vi "RT Driver VI.vi"(6 "Device Clock":string, 9 "Device Inputs FIFO":refnum<k33>, 10 "Device Outputs FIFO":refnum<k33>, 11 "Device Reference":T1 format="%.0x") -> ()   [LabVIEW 2019, in "Displacement Measurement CD Engine.lvlib"]
uses:
  Displacement Measurement CD Engine.lvlib
  <vilib>/NI VeriStand/Custom Device API/Custom Device Item Ref.ctl
  <vilib>/NI VeriStand/Custom Device API/Custom Device Channel Type.ctl
  <vilib>/NI VeriStand/Custom Device API/Message Response (String).ctl
  <vilib>/NI VeriStand/Custom Device API/Message Response (Byte Array).ctl
  <vilib>/DAQmx/read.llb/DAQmx Read (Analog 2D DBL NChan NSamp).vi
  <vilib>/NI VeriStand/Custom Device API/Get Item Property (Double).vi
  <vilib>/NI VeriStand/Custom Device API/Get Item Property (String).vi
  <vilib>/DAQmx/create/channels.llb/DAQmx Create Channel (AI-Voltage-Basic).vi
  <vilib>/DAQmx/configure/timing.llb/DAQmx Timing (Sample Clock).vi
  <vilib>/DAQmx/miscellaneous.llb/DAQmx Fill In Error Info.vi
  <vilib>/NI VeriStand/Custom Device API/Custom Device API.lvlib
  <vilib>/NI VeriStand/Custom Device Tools/Custom Device Utility Library/Custom Device Utility Library.lvlib
  <resource>/objmgr/daqmx.rc
panel:
  in  "Initialization Status Notifier":refnum<notifier>
  in  "Status Notifier":refnum<notifier>
  # "Custom Device Template\nv1.0"
  # "Use this template as a starting point for creating a custom device code module. The input controls shown here are specially named controls that the system will use to provide the device loop with data. The controls are not required for the device loop to run. For instance, if the device doesn't produce any output data, then you don't need the Device Outputs FIFO control. If you do use these controls, however, they need to have these exact names to be functional."
  # "The optional status notifier element is used to notify the RT engine of the last state of the custom device, and to indicate the device has completed execution. If this control is not used, a default No Error value is returned to the system when the device finishes execution.\n\nNote: This error state is not checked until the system shuts down. Use an output status channel to send more immediate status values to the system."
  # "This optional input can be used to send the VeriStand Engine the final status of the custom device initalization process. If this control exists on the custom device front panel, the VeriStand Engine will wait for a status update before starting up. If the custom device reports an error, that will abort the execution of the current configuration in the VeriStand Engine.\n\nThis control can be deleted if the custom device does not need to send the initialization status update."
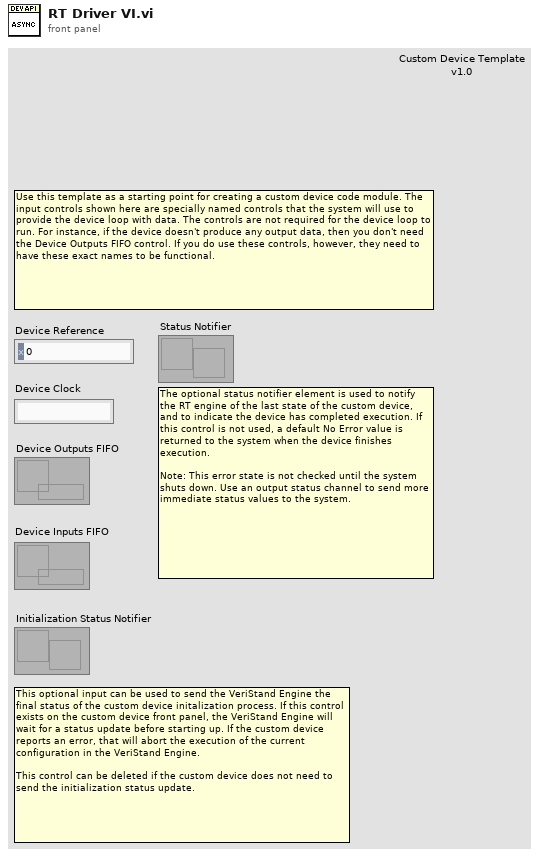
[diagram p1: front panel]
types:
  T1 = typedef "Custom Device API.lvlib/Custom Device Item Ref.ctl" = u64
  T2 = typedef "Custom Device API.lvlib/Custom Device Channel Type.ctl" = enum16{"Input", "Output"}
  T3 = typedef "Custom Device API.lvlib/Custom Device Engine Event Ref.ctl" = refnum<event-registration>
  T4 = typedef "Custom Device API.lvlib/Message Response (String).ctl" = cluster{"Response":string, "Error":errorcluster}
  T5 = typedef "Custom Device API.lvlib/Message Response (Byte Array).ctl" = cluster{"Response":u8[], "Error":errorcluster}
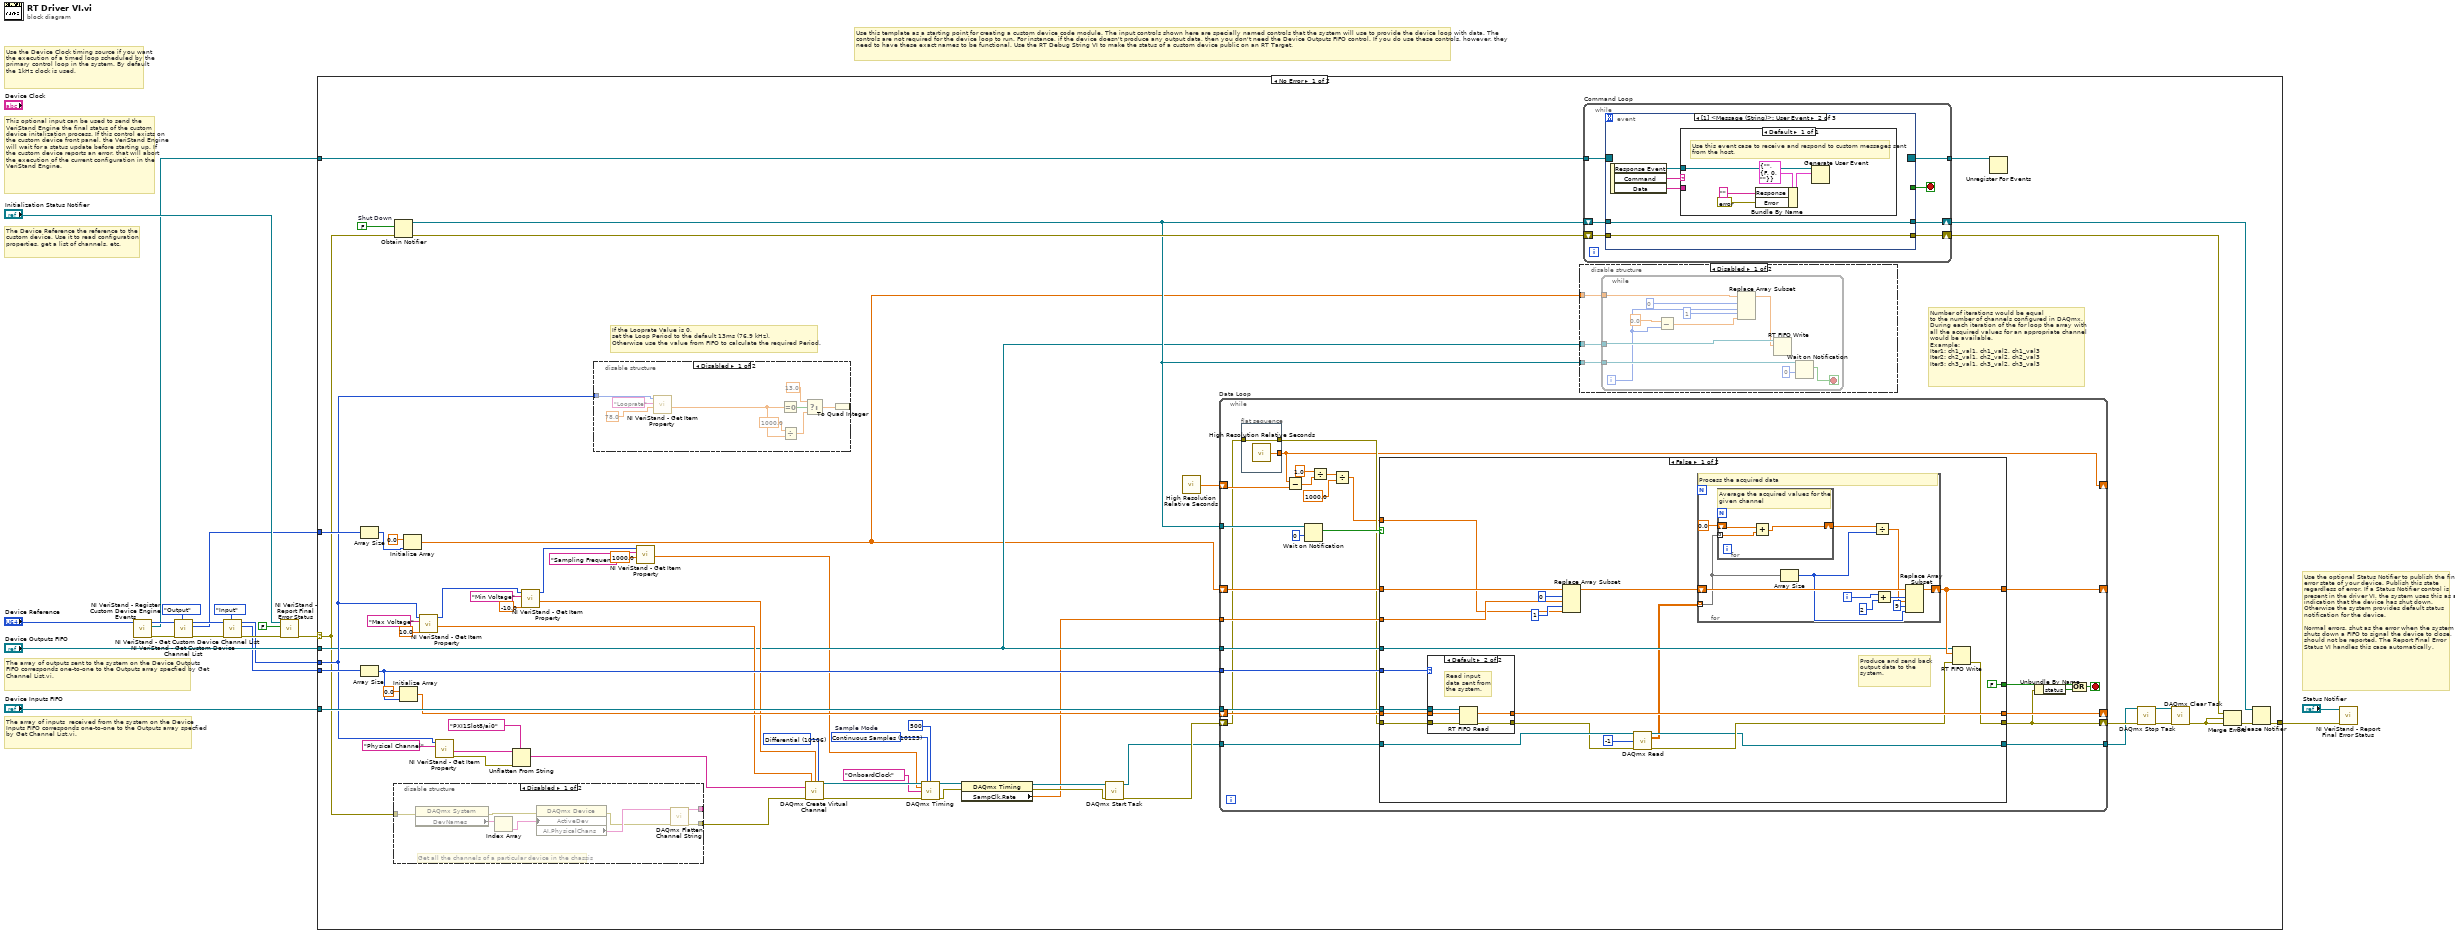
[diagram p0: block diagram]
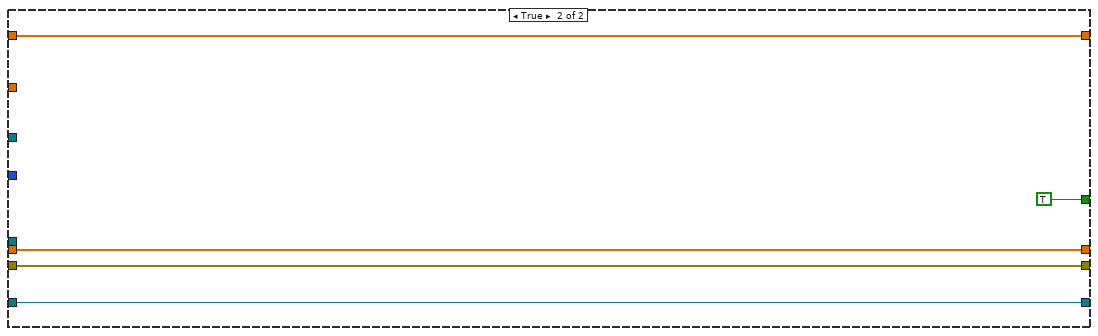
[diagram p4: hidden frame]
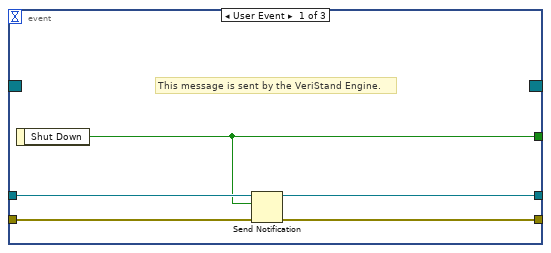
[diagram p7: hidden frame]
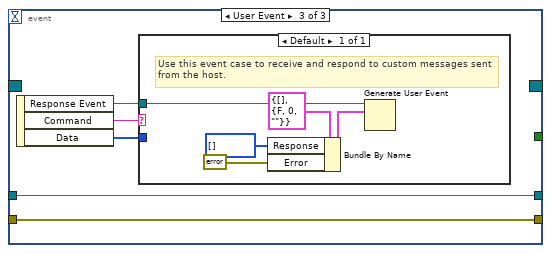
[diagram p8: hidden frame]
diagram:
  # "This optional input can be used to send the VeriStand Engine the final status of the custom device initalization process. If this control exists on the custom device front panel, the VeriStand Engine will wait for a status update before starting up. If the custom device reports an error, that will abort the execution of the current configuration in the VeriStand Engine."
  # "The array of inputs  received from the system on the Device Inputs FIFO corresponds one-to-one to the Outputs array specfied by Get Channel List.vi."
  # "Use the optional Status Notifier to publish the final error state of your device. Publish this state regardless of error. If a Status Notifier control is present in the driver VI, the system uses this as an indication that the device has shut down. Otherwise the system provides default status notification for the device.\n\nNormal errors, shut as the error when the system shuts down a FIFO to signal the device to close, should not be reported. The Report Final Error Status VI handles this case automatically."
  # "The array of outputs sent to the system on the Device Outputs FIFO corresponds one-to-one to the Outputs array specfied by Get Channel List.vi."
  # "The Device Reference the reference to the custom device. Use it to read configuration properties, get a list of channels, etc."
  # "Use the Device Clock timing source if you want the execution of a timed loop scheduled by the primary control loop in the system. By default the 1kHz clock is used."
  # "Use this template as a starting point for creating a custom device code module. The input controls shown here are specially named controls that the system will use to provide the device loop with data. The controls are not required for the device loop to run. For instance, if the device doesn't produce any output data, then you don't need the Device Outputs FIFO control. If you do use these controls, however, they need to have these exact names to be functional. Use the RT Debug String VI to make the status of a custom device public on an RT Target."
  n1 = call <vilib>:"NI VeriStand - Register Custom Device Engine Events.vi"("Device Ref in"="Device Reference") -> ("error out"=w19:errorcluster, "Custom Device Engine Event Ref"=w4:T3, "Device Ref out"=w10:T1)  [unwired: 8 in]
  n2 = call <vilib>:"NI VeriStand - Get Custom Device Channel List.vi"("Channel Type"=Custom_Device_Channel_Type."Output", "error in (no error)"=w19, "Device Ref in"=w10) -> ("error out"=w14:errorcluster, "Specified Channel Ref List"=w3:T1[], "Device Ref out"=w15:T1)  [unwired: 6 out]
  n3 = call <vilib>:"NI VeriStand - Get Custom Device Channel List.vi"("Channel Type"=Custom_Device_Channel_Type."Input", "error in (no error)"=w14, "Device Ref in"=w15) -> ("error out"=w18:errorcluster, "Specified Channel Ref List"=w6:T1[], "Device Ref out"=w2:T1)  [unwired: 6 out]
  n4 = call <vilib>:"NI VeriStand - Report Final Error Status.vi"("error in (no error)"=w18, "Filter FIFO & Shutdown Errors (T)"=FALSE ("Filter FIFO Errors (T)"), "Status Notifier"="Initialization Status Notifier") -> ("error out"=w1:errorcluster)  [unwired: 8 out]
  n5 = case shown="No Error" w1 {
    selector: w1 -> [w28 w215]
    tunnel: "Device Outputs FIFO" -> [w34 _]
    tunnel: "Device Inputs FIFO" -> [w75 _]
    tunnel: w6 -> [w71 _]
    tunnel: w3 -> [w70 _]
    tunnel: w4 -> [w68 _]
    tunnel: [w66 w215] -> w5
    tunnel: w2 -> [w43 _]
    frame No Error {
      w49 = 10106 items=["default"=-1, "RSE"=10083, "NRSE"=10078, "Differential"=10106, "Pseudodifferential"=12529] ("Terminal Configuration")
      w51 = 10123 items=["Finite Samples"=10178, "Continuous Samples"=10123, "Hardware Timed Single Point"=12522]  # Sample Mode
      w67 = FALSE  # Shut Down
      # "Number of iterations would be equal\nto the number of channels configured in DAQmx.\nDuring each iteration of the for loop the array with\nall the acquired values for an appropriate channel\nwould be available.\nExample:\nIter1: ch1_val1, ch1_val2, ch1_val3\nIter2: ch2_val1, ch2_val2, ch2_val3\nIter3: ch3_val1, ch3_val2, ch3_val3"
      # "If the Looprate Value is 0,\nset the Loop Period to the default 13ms (76.9 kHz).\nOtherwise use the value from FIFO to calculate the required Period."
      n6 = Array Size(array=w71) -> (size(s)=w69:i32)
      n7 = Array Size(array=w70) -> (size(s)=w72:i32)
      n8 = disable-structure shown="Disabled" {
        disable-tunnel: [w166 _] -> _
        disable-tunnel: w28 -> [w164 _]
        disable-tunnel: [w161 _] -> w27
        frame Disabled {
          # "Get all the channels of a particular device in the chassis"
          n9 = property class="DAQmx System"(error in=w164) -> (error out=w163:errorcluster, "DevNames"=w168:tag[])  [unwired: 1 in, 1 out]
          n10 = Index Array(array=w168) -> (element=w167:tag)  [unwired: 1 in]
          n11 = property class="DAQmx Device"(error in=w163, "ActiveDev"=w167) -> (error out=w162:errorcluster, "AI.PhysicalChans"=w165:tag[])  [unwired: 1 in, 1 out]
          n12 = call <vilib>:"DAQmx Flatten Channel String.vi"("names in"=w165, "error in"=w162) -> ("names out"=w166:string, "error out"=w161:errorcluster)  [unwired: 12 in]
        }
        frame Enabled {
        }
      }
      n13 = Obtain Notifier(notification data type=w67, error in (no error)=w28) -> (notifier out=w35:refnum<notifier>, error out=w76:errorcluster)  [unwired: 2 in, 1 out]
      n14 = Initialize Array(0.0 ("element"), w69) -> (w62:dbl[])
      n15 = Initialize Array(0.0 ("element"), w72) -> (w33:dbl[])
      n16 = call-poly <vilib>:"NI VeriStand - Get Item Property.vi"("Default Value"=10.0, "Property Name"="Max Voltage", "Item Ref in"=w43) -> ("Value"=w41:dbl, "Item Ref out"=w42:T1)  [unwired: 5 in, 2 out]
      n17 = call-poly <vilib>:"NI VeriStand - Get Item Property.vi"("Property Name"="Physical Channel", "Item Ref in"=w43) -> ("error out"=w45:errorcluster, "Value"=w29:string)  [unwired: 6 in, 2 out]
      n18 = Unflatten From String(type=tag "PXI1Slot8/ai0" ("Physical Channel"), binary string=w29, error in (no error)=w45) -> (value=w24:tag)  [unwired: 2 in, 2 out]
      n19 = call-poly <vilib>:"NI VeriStand - Get Item Property.vi"("Default Value"=-10.0, "Property Name"="Min Voltage", "Item Ref in"=w42) -> ("Value"=w40:dbl, "Item Ref out"=w44:T1)  [unwired: 5 in, 2 out]
      n20 = disable-structure shown="Disabled" {
        disable-tunnel: w43 -> [w79 _]
        frame Disabled {
          n21 = call-poly <vilib>:"NI VeriStand - Get Item Property.vi"("Default Value"=78.0, "Property Name"="Looprate", "Item Ref in"=w79) -> ("Value"=w77:dbl)  [unwired: 5 in, 3 out]
          n22 = Equal To 0?(x=w77) -> (x = 0?=w84:bool)
          n23 = Divide(x=1000.0, y=w77) -> (x/y=w82:dbl)
          n24 = Select(t=13.0, s=w84, f=w82) -> (s? t:f=w81:dbl)
          n25 = To Quad Integer(1:w81) -> ()  [unwired: 1 out]
        }
        frame Enabled {
        }
      }
      n26 = call-poly <vilib>:"NI VeriStand - Get Item Property.vi"("Default Value"=1000.0, "Property Name"="Sampling Frequency", "Item Ref in"=w44) -> ("Value"=w23:dbl)  [unwired: 5 in, 3 out]
      n27 = call-poly <vilib>:"DAQmx Create Virtual Channel.vi"("maximum value"=w41, "minimum value"=w40, "input terminal configuration"=w49, "physical channels"=w24, "error in"=w27) -> ("task out"=w50:refnum<k21>, "error out"=w30:errorcluster)  [unwired: 9 in]
      n28 = call-poly <vilib>:"DAQmx Timing.vi"("task/channels in"=w50, "sample mode"=w51, "samples per channel"=500, "rate"=w23, "source"=tag "OnboardClock" ("Sample Clock Source"), "error in"=w30) -> ("task out"=w53:refnum<k21>, "error out"=w52:errorcluster)  [unwired: 8 in]
      n29 = property class="DAQmx Timing"(reference=w53, error in=w52) -> (reference out=w47:refnum<k21>, error out=w46:errorcluster, "SampClk.Rate"=w22:dbl)
      n30 = call <vilib>:"DAQmx Start Task.vi"("task/channels in"=w47, "error in"=w46) -> ("task out"=w25:refnum<k21>, "error out"=w26:errorcluster)  [unwired: 12 in]
      n31 = call <vilib>:"High Resolution Relative Seconds.vi"() -> ("relative seconds"=w21:dbl)
      n32 = while "Data Loop" {
        shift-right: [w110] -> _
        shift-left: w62 -> [w111]
        shift-right: [w105] -> w59
        shift-left: w26 -> [w93]
        shift-right: [w109] -> _
        shift-left: w33 -> [w97]
        tunnel: w34 -> [w96]
        tunnel: w75 -> [w108]
        tunnel: w69 -> [w107]
        tunnel: w35 -> [w104]
        tunnel: w25 -> [w99]
        tunnel: [w98] -> w58
        tunnel: w22 -> [w95]
        shift-right: [w91] -> _
        shift-left: w21 -> [w94]
        stop <- w100 stop-if-true
        n33 = flat-sequence {
          tunnel: w93 -> [w113]
          tunnel: [w113] -> w92
          tunnel: [w112] -> w91
          frame #0 {
            n34 = call <vilib>:"High Resolution Relative Seconds.vi"() -> ("relative seconds"=w112:dbl)
          }
        }
        n35 = Subtract(x=w91, y=w94) -> (x-y=w89:dbl)
        n36 = Wait on Notification(notifier=w104, timeout in ms (-1)=0) -> (notification=w103:bool)  [unwired: 2 in, 3 out]
        n37 = Divide(x=1.0, y=w89) -> (x/y=w88:dbl)
        n38 = Divide(x=w88, y=1000.0) -> (x/y=w86:dbl)
        n39 = case shown="False" w103 {
          tunnel: w92 -> [w134 w159]
          tunnel: w111 -> [w133 w160]
          tunnel: [w132 w160] -> w110
          tunnel: w97 -> [w122 w158]
          tunnel: [w119 w158] -> w109
          tunnel: w96 -> [w118 _]
          tunnel: w108 -> [w131 _]
          tunnel: w107 -> [w130 _]
          tunnel: [w129 w159] -> w105
          tunnel: [FALSE TRUE] -> w101
          tunnel: w99 -> [w128 w156]
          tunnel: [w125 w156] -> w98
          tunnel: w95 -> [w117 _]
          tunnel: w86 -> [w115 _]
          frame False {
            # "Produce and send back output data to the system."
            n40 = case shown="Default" w130 {
              tunnel: w131 -> [_ w155]
              tunnel: w133 -> [w150 w154]
              tunnel: [w150 w153] -> w132
              tunnel: [w149 w152] -> w127
              tunnel: w134 -> [w149 w151]
              frame 0 {
                # "No inputs to read\nfrom system. Inputs FIFO not created in this case, so don't write to it."
              }
              frame Default {
                # "Read input data sent from the system."
                n41 = RT FIFO Read(0:w155, 1:w154, 3:w151) -> (9:w153:dbl[], 11:w152:errorcluster)  [unwired: 4 out]
              }
            }
            n42 = Replace Array Subset(array=w122, new element #1=w117, index #1=0 ("index"), new element #2=w115, index #2=1 ("index")) -> (w120:dbl[])
            n43 = call-poly <vilib>:"DAQmx Read.vi"("task/channels in"=w128, "number of samples per channel"=-1, "error in"=w127) -> ("task out"=w125:refnum<k21>, "data"=w114:dbl[][], "error out"=w126:errorcluster)  [unwired: 10 in]
            n44 = for {
              shift-right: [w144] -> w119
              shift-left: w120 -> [w145]
              tunnel: w114 -> [w137] mode=indexing
              i -> [w143]
              # "Process the acquired data"
              n45 = for {
                tunnel: w137 -> [w147] mode=indexing
                shift-right: [w146] -> w139
                shift-left: 0.0 -> [w148]
                # "Average the acquired values for the given channel"
                n46 = Add(x=w148, y=w147) -> (x+y=w146:dbl)
              }
              n47 = Array Size(array=w137) -> (size(s)=w135:i32)
              n48 = Divide(x=w139, y=w135) -> (x/y=w138:dbl)
              n49 = Add(x=w143, y=2) -> (x+y=w141:i32)
              n50 = Replace Array Subset(array=w145, new element #1=w138, index #1=w141, new element #2=w135, index #2=9 ("index")) -> (w144:dbl[])
            }
            n51 = RT FIFO Write(0:w118, 1:w119, 3:w126) -> (11:w129:errorcluster)  [unwired: 1 in, 4 out]
          }
          frame True {
          }
        }
        n52 = Unbundle By Name(w105) -> ("status"=w102:bool)
        n53 = Compound Arithmetic op=OR(w101, w102) -> (w100:bool)
      }
      n54 = disable-structure shown="Disabled" {
        disable-tunnel: w35 -> [w171 _]
        disable-tunnel: w34 -> [w170 _]
        disable-tunnel: w33 -> [w169 _]
        frame Disabled {
          n55 = while {
            tunnel: w171 -> [w180]
            tunnel: w170 -> [w179]
            tunnel: w169 -> [w177]
            i -> [w174]
            stop <- w181 stop-if-true
            n56 = Subtract(x=0.0, y=w174) -> (x-y=w173:dbl)
            n57 = Replace Array Subset(array=w177, new element #1=w174, index #1=0 ("index"), new element #2=w173, index #2=1 ("index")) -> (w176:dbl[])
            n58 = RT FIFO Write(0:w179, 1:w176) -> ()  [unwired: 2 in, 5 out]
            n59 = Wait on Notification(notifier=w180, timeout in ms (-1)=0) -> (notification=w181:bool)  [unwired: 2 in, 3 out]
          }
        }
        frame Enabled {
        }
      }
      n60 = while "Command Loop" {
        tunnel: w68 -> [w189]
        tunnel: [w188] -> w65
        shift-right: [w185] -> w64
        shift-left: w35 -> [w186]
        shift-right: [w183] -> w39
        shift-left: w76 -> [w184]
        stop <- w187 stop-if-true
        n61 = event shown="[1] <Message (String)>: User Event" {
          selector: w189 -> [_ _ _]
          dyn-events: [_ _ _] -> w188
          timeout: _ -> [_ _ _]
          tunnel: [w192 _ _] -> w187
          tunnel: w186 -> [w193 w197 w207]
          tunnel: [w194 w197 w207] -> w185
          tunnel: w184 -> [w191 w195 w205]
          tunnel: [w190 w195 w205] -> w183
          event User Event {
            # "This message is sent by the VeriStand Engine."
            n62 = event-data() -> ("Shut Down"=w192:bool)  [unwired: 1 in]
            n63 = Send Notification(notification=w192, notifier=w193, error in (no error)=w191) -> (notifier out=w194:refnum<notifier>, error out=w190:errorcluster)
          }
          event User Event {
            n64 = event-data() -> ("Response Event"=w196:refnum<user-event>, "Command"=w199:string, "Data"=w198:string)  [unwired: 1 in]
            n65 = case shown="Default" w199 {
              tunnel: w198 -> [_]
              tunnel: w196 -> [w204]
              frame Default {
                # "Use this event case to receive and respond to custom messages sent from the host."
                n66 = Bundle By Name(cluster=T4 {"Response"="", "Error"={"status"=FALSE, "code"=0, "source"=""}} ("event data"), "Response"="", "Error"=errorcluster {"status"=FALSE, "code"=0, "source"=""}) -> (w202:T4)
                n67 = Generate User Event(user event=w204, event data cluster=w202) -> ()  [unwired: 2 in, 2 out]
              }
            }
          }
          event User Event {
            n68 = event-data() -> ("Response Event"=w206:refnum<user-event>, "Command"=w209:string, "Data"=w208:u8[])  [unwired: 1 in]
            n69 = case shown="Default" w209 {
              tunnel: w208 -> [_]
              tunnel: w206 -> [w214]
              frame Default {
                # "Use this event case to receive and respond to custom messages sent from the host."
                n70 = Bundle By Name(cluster=T5 {"Response"=[], "Error"={"status"=FALSE, "code"=0, "source"=""}} ("event data"), "Response"=u8[] [], "Error"=errorcluster {"status"=FALSE, "code"=0, "source"=""}) -> (w211:T5)
                n71 = Generate User Event(user event=w214, event data cluster=w211) -> ()  [unwired: 2 in, 2 out]
              }
            }
          }
        }
      }
      n72 = Unregister For Events(event registration refnum=w65) -> ()  [unwired: 1 in, 1 out]
      n73 = call <vilib>:"DAQmx Stop Task.vi"("task/channels in"=w58, "error in"=w59) -> ("task out"=w60:refnum<k21>, "error out"=w61:errorcluster)  [unwired: 12 in]
      n74 = call <vilib>:"DAQmx Clear Task.vi"("task in"=w60, "error in"=w61) -> ("error out"=w32:errorcluster)  [unwired: 13 in]
      n75 = Merge Errors(w39, w32, w32) -> (w63:errorcluster)
      n76 = Release Notifier(notifier=w64, error in (no error)=w63) -> (error out=w66:errorcluster)  [unwired: 1 in, 2 out]
    }
    frame Error {
    }
  }
  n77 = call <vilib>:"NI VeriStand - Report Final Error Status.vi"("error in (no error)"=w5, "Status Notifier"="Status Notifier") -> ()  [unwired: 1 in, 9 out]
